vi "Shutdown.vi"(8 "error in":errorcluster, 11 "Camera in":refnum<class "Camera.lvclass">) -> (0 "error out":errorcluster, 3 "Camera out":refnum<class "Camera.lvclass">)   [LabVIEW 2018, in "Camera.lvlib" / "Camera.lvclass"]
uses:
  Camera.lvclass
  Camera.lvclass/Camera.ctl
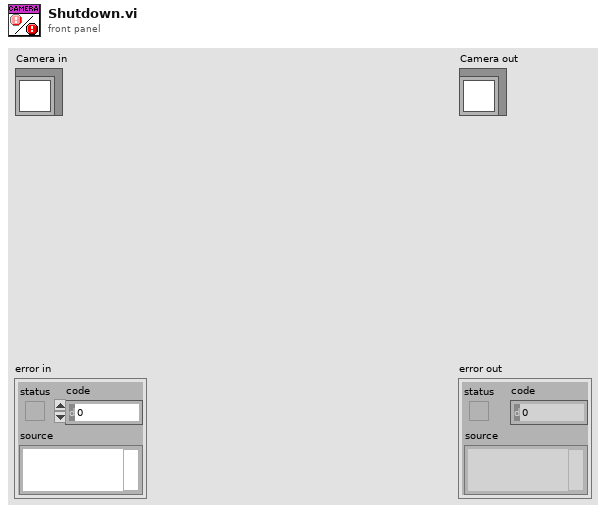
[diagram p1: front panel]
types:
  T1 = typedef "IMAQ Image.ctl" = refnum<image>
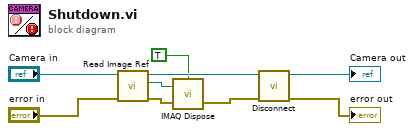
[diagram p0: block diagram]
diagram:
  n1 = call "Read Image Ref.vi"("error in (no error)"="error in", "Camera in"="Camera in") -> ("error out"=w6:errorcluster, "Image"=w7:T1, "Camera out"=w2:refnum<class "Camera.lvclass">)  [unwired: 7 in]
  n2 = call "IMAQ Dispose"("All Images? (No)"=TRUE, "Image"=w7, "error in (no error)"=w6) -> ("error out"=w4:errorcluster)  [unwired: 3 in]
  n3 = call-dynamic "Disconnect.vi"("error in (no error)"=w4, "Camera in"=w2) -> ("error out"=→"error out":errorcluster, "Camera out"=→"Camera out":refnum<class "Camera.lvclass">)  [unwired: 8 in]
